vi "Configure.vi"(8 "error in (no error)":errorcluster, 10 "Configuration":refnum<class "Column Configuration.lvclass">, 11 "Composed Column Factory in":refnum<class "Composed Column Factory.lvclass">) -> (0 "error out":errorcluster, 3 "Composed Column Factory out":refnum<class "Composed Column Factory.lvclass">)   [LabVIEW 2020, in "Composed Columns.lvlib" / "Composed Column Factory.lvclass"]
uses:
  Composed Column Factory.lvclass
  Basic Columns/Column Configuration/Basic Column Configuration Class/Column Configuration.lvclass
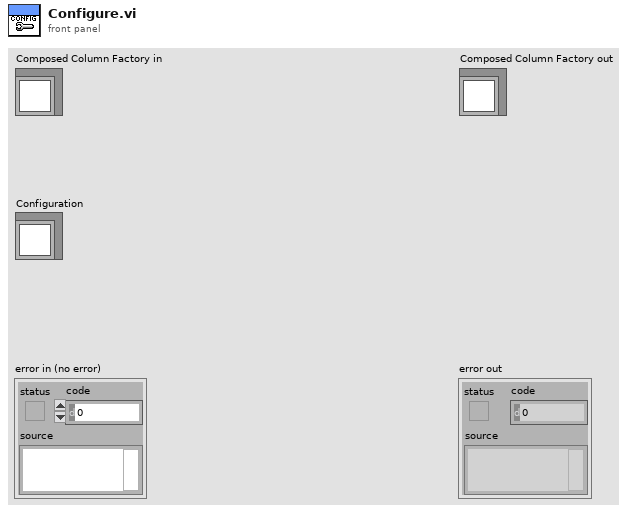
[diagram p1: front panel]
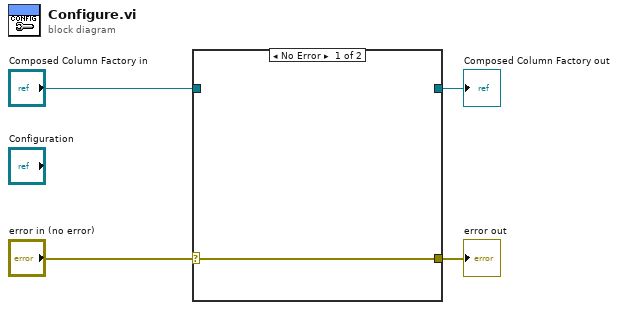
[diagram p0: block diagram]
diagram:
  n1 = case shown="No Error" "error in (no error)" {
    selector: "error in (no error)" -> [w5 w7]
    tunnel: [w5 w7] -> w3
    tunnel: "Composed Column Factory in" -> [_ w6]
    tunnel: [_ w6] -> w1
    frame No Error {
    }
    frame Error {
    }
  }
  "error out" <- w3
  "Composed Column Factory out" <- w1
